vi "CLD 7 Time Stamp to String Challenge Exercise.vi"(8 "Error In":errorcluster) -> (0 "Error Out":errorcluster, 3 "Code String Out":string)   [LabVIEW 2009]
doc: "CLD 7 exercise"
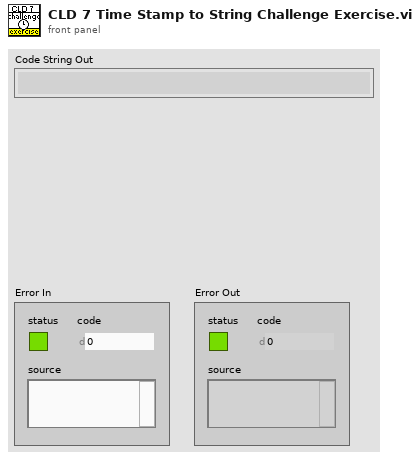
[diagram p1: front panel]
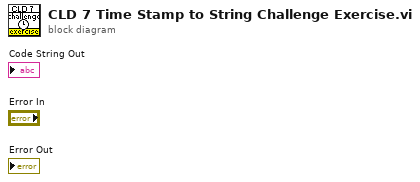
[diagram p0: block diagram]
diagram:
